vi "randgen.vi"() -> ()   [LabVIEW 2018]
panel:
  out "output of last iteration":dbl
  in  "stop":bool
  out "Average of recent 5 values.":dbl
  out "Value of Previous iteration":dbl
  out "iterate through array \nin another for loop":dbl
  out "Min Value Index":dbl
  out "Min Value":dbl
  out "Max Value Index":dbl
  out "Max Value":dbl
  out "Data at array index":dbl
  in  "index of array":dbl
  out "Array SIze":dbl
  out "Array":dbl[](array[numeric])
  in  "wait time in ms":dbl
  out "Current Loop Iteration":dbl
  in  "For Loops Iteration times":dbl
  out "Random Num":dbl
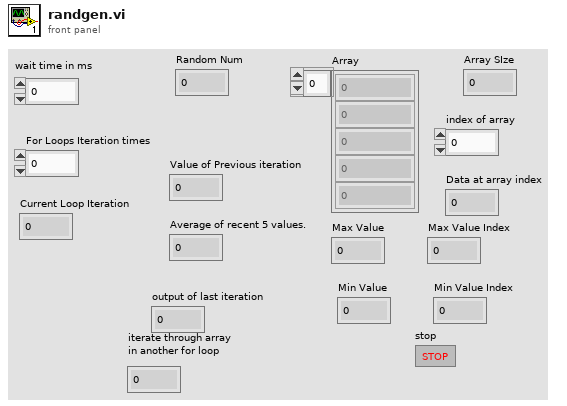
[diagram p1: front panel]
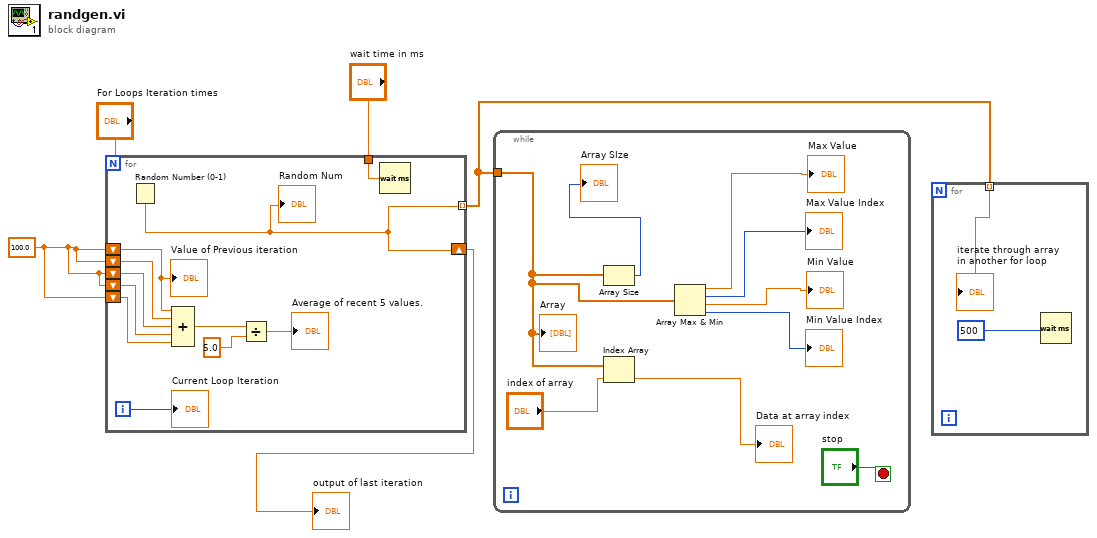
[diagram p0: block diagram]
diagram:
  w1 = 100.0 ("number: 0 to 1")
  n1 = for {
    N: "For Loops Iteration times" -> [_]
    tunnel: "wait time in ms" -> [w15]
    tunnel: [w6] -> w3 mode=indexing
    shift-right: [w6] -> w2
    shift-left: w1 -> [w14]
    shift-left: w1 -> [w13]
    shift-left: w1 -> [w12]
    shift-left: w1 -> [w11]
    shift-left: w1 -> [w10]
    i -> [w16]
    n2 = Random Number (0-1)() -> (number: 0 to 1=w6:dbl)
    "Random Num" <- w6
    n3 = Compound Arithmetic op=ADD(w14, w13, w12, w11, w10) -> (w8:dbl)
    n4 = Divide(x=w8, y=5.0) -> (x/y=→"Average of recent 5 values.":dbl)
    n5 = Wait (ms)(milliseconds to wait=w15) -> ()  [unwired: 1 out]
    "Current Loop Iteration" <- w16
    "Value of Previous iteration" <- w14
  }
  "output of last iteration" <- w2
  n6 = while {
    tunnel: w3 -> [w18]
    stop <- "stop" stop-if-true
    n7 = Array Size(array=w18) -> (size(s)=→"Array SIze":i32)
    n8 = Index Array(array=w18, index="index of array") -> (element=→"Data at array index":dbl)
    n9 = Array Max & Min(array=w18) -> (max value=→"Max Value":dbl, max index (indices)=→"Max Value Index":i32, min value=→"Min Value":dbl, min index (indices)=→"Min Value Index":i32)
    "Array" <- w18
  }
  n10 = for {
    tunnel: w3 -> [w27] mode=indexing
    n11 = Wait (ms)(milliseconds to wait=u32 500) -> ()  [unwired: 1 out]
    "iterate through array \nin another for loop" <- w27
  }
